vi "SysInfo-Get Version Info.vi"() -> (4 "folder":path, 6 "version":string, 8 "formatted version":string)   [LabVIEW 2020]
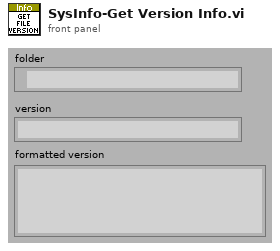
[diagram p1: front panel]
types:
  T1 = cluster{"Major":i32, "Minor":i32, "Build":i32, "Private":i32, "FileVersion":string, "ProductName":string, "InternalName":string, "CompanyName":string, "LegalCopyright":string, "FileDescription":string}
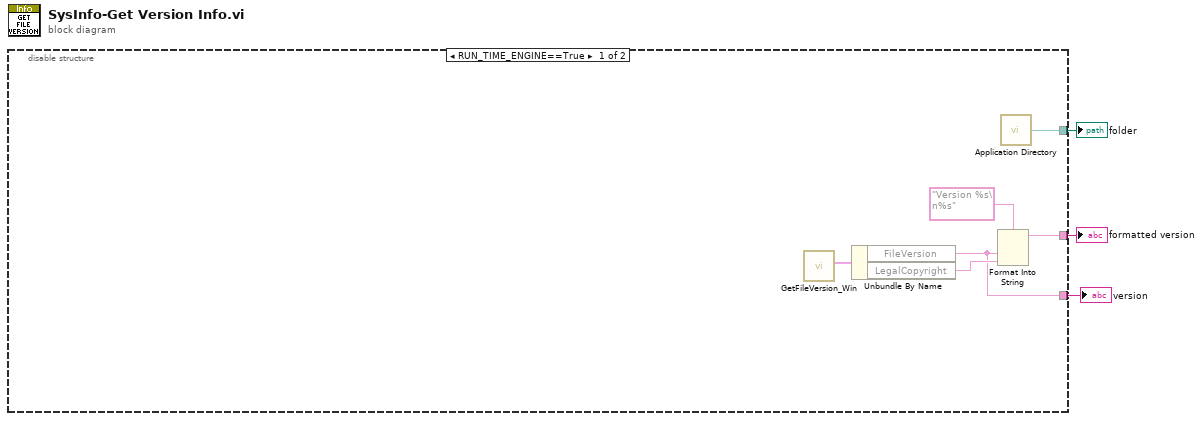
[diagram p0: block diagram]
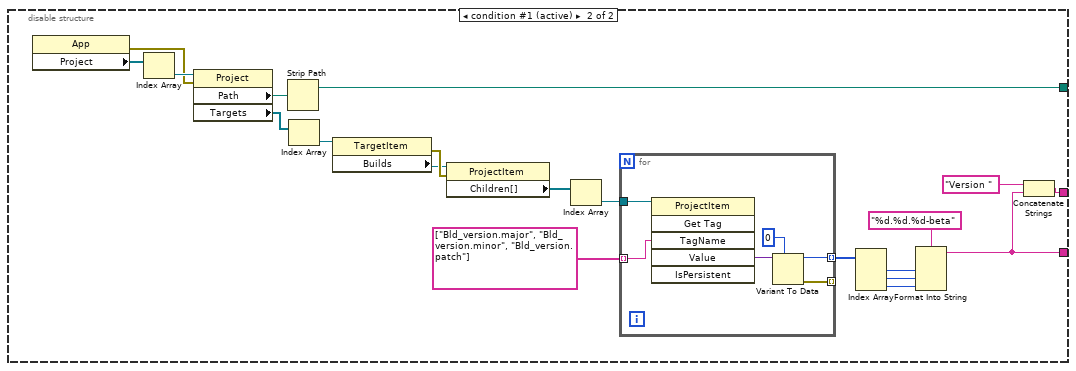
[diagram p2: hidden frame]
diagram:
  n1 = disable-structure shown="RUN_TIME_ENGINE==True" {
    disable-tunnel: [w7 w29] -> w3
    disable-tunnel: [w5 w23] -> w2
    disable-tunnel: [w4 w10] -> w1
    frame condition #0 {
      n2 = call "GetFileVersion_Win.vi"() -> ("File Info Out"=w8:T1)  [unwired: 9 in, 2 out]
      n3 = Unbundle By Name(w8) -> ("FileVersion"=w4:string, "LegalCopyright"=w6:string)
      n4 = Format Into String(format string="Version %s\n%s", w4, w6) -> (resulting string=w7:string)  [unwired: 2 in, 1 out]
      n5 = call <vilib>:"Application Directory.vi"() -> ("Application Directory"=w5:path)
    }
    frame condition #1 (active) {
      n6 = property class="App"() -> (error out=w25:errorcluster, "Project"=w26:refnum<vi>[])  [unwired: 2 in, 1 out]
      n7 = Index Array(array=w26) -> (element=w27:refnum<vi>)  [unwired: 1 in]
      n8 = property class="Project"(reference=w27, error in=w25) -> ("Path"=w24:path, "Targets"=w19:refnum<vi>[])  [unwired: 2 out]
      n9 = Strip Path(path=w24) -> (stripped path=w23:path)  [unwired: 1 out]
      n10 = Index Array(array=w19) -> (element=w21:refnum<vi>)  [unwired: 1 in]
      n11 = property class="TargetItem"(reference=w21) -> (error out=w22:errorcluster, "Builds"=w20:refnum<vi>)  [unwired: 1 in, 1 out]
      n12 = property class="ProjectItem"(reference=w20, error in=w22) -> ("Children[]"=w18:refnum<vi>[])  [unwired: 2 out]
      n13 = Index Array(array=w18) -> (element=w17:refnum<vi>)  [unwired: 1 in]
      n14 = for {
        tunnel: w17 -> [w35]
        tunnel: string[] ["Bld_version.major", "Bld_version.minor", "Bld_version.patch"] -> [w34] mode=indexing
        tunnel: [w31] -> w15 mode=indexing
        tunnel: [w30] -> _ mode=indexing
        n15 = invoke class="ProjectItem" method="Get Tag"(reference=w35, "TagName"=w34) -> ("Value"=w33:variant)  [unwired: 4 in, 5 out]
        n16 = Variant To Data(type=0, Variant=w33) -> (data=w31:i32, error out=w30:errorcluster)  [unwired: 1 in]
      }
      n17 = Index Array(array=w15) -> (element #1=w13:i32, element #2=w12:i32, element #3=w11:i32)  [unwired: 3 in]
      n18 = Format Into String(format string="%d.%d.%d-beta", w13, w12, w11) -> (resulting string=w10:string)  [unwired: 2 in, 1 out]
      n19 = Concatenate Strings("Version ", w10) -> (w29:string)
    }
  }
  "formatted version" <- w3
  "folder" <- w2
  "version" <- w1
